vi "read_db.vi"(8 "error in (no error)":errorcluster, 11 "Constraints":T4={"Upper Timestamp Range"=timestamp(0 s since 1904-01-01), "Lower Timestamp Range"=timestamp(0 s since 1904-01-01), "Experiment Group:"="", "Experiment Name:"=[], "Upper Velocity Limit (km/s)"=0.0, "Lower Velocity Limit (km/s)"=0.0, "Upper Mass Limit (kg)"=0.0, "Lower Mass Limit (kg)"=0.0, "Estimate Source "=-2, "name array"=[]} {"Estimate Source" items=["Any Source."=-2, "No Shot"=-1, "Basic Labview Estimate"=0, "IDL Estimate From Andrew"=1, "IDL Estimate From Tobin"=2, "Old Metadata"=3]; "Lower Mass Limit (kg)" min=-1.0 max=1.0 step=1e-20; "Upper Mass Limit (kg)" min=-1.0 max=1.0 step=1e-20; "Lower Velocity Limit (km/s)" min=-1.0 max=299792000.0; "Upper Velocity Limit (km/s)" min=-1.0 max=299792000.0}) -> (0 "error out":errorcluster, 1 "Experiment Settings ID Array":i64[](array[numeric]), 2 "Dust Event ID Array":i64[](array[numeric]), 3 "Dust Array":T1[](array[typedef]) {"File Location" items=["Currently Writing"=-3, "Labview Files"=-2, "Mars Data Processing Factility"=-1, "Local Cache "=0, "Old Storage"=1, "Storage"=2]; "Estimate Source" items=["Any Source."=-2, "No Shot"=-1, "Basic Labview Estimate"=0, "IDL Estimate From Andrew"=1, "IDL Estimate From Tobin"=2, "Old Metadata"=3]}, 5 "File Location Array":i64[](array[numeric]))   [LabVIEW 2012]
uses:
  Constraints.ctl
  Estimate_source.ctl
  Public API/Query_Dust_Event.ctl
  File_location.ctl
  <vilib>/addons/database/Auxilliary.llb/DB Tools Cursor Type.ctl
  <vilib>/addons/database/Connection.llb/Conn Execute.vi
  <vilib>/addons/database/Recordset.llb/Rec Fetch Recordset Data (R).vi
  <vilib>/addons/database/Recordset.llb/Rec Destroy - Connection.vi
  <vilib>/addons/database/_DB Variant To Data/Database Variant To Data.xnode
  <vilib>/addons/database/NI_Database_API.lvlib
panel:
  out "concatenated string":string
  out "SQL Query Sintax":string
  # "Dust Event"
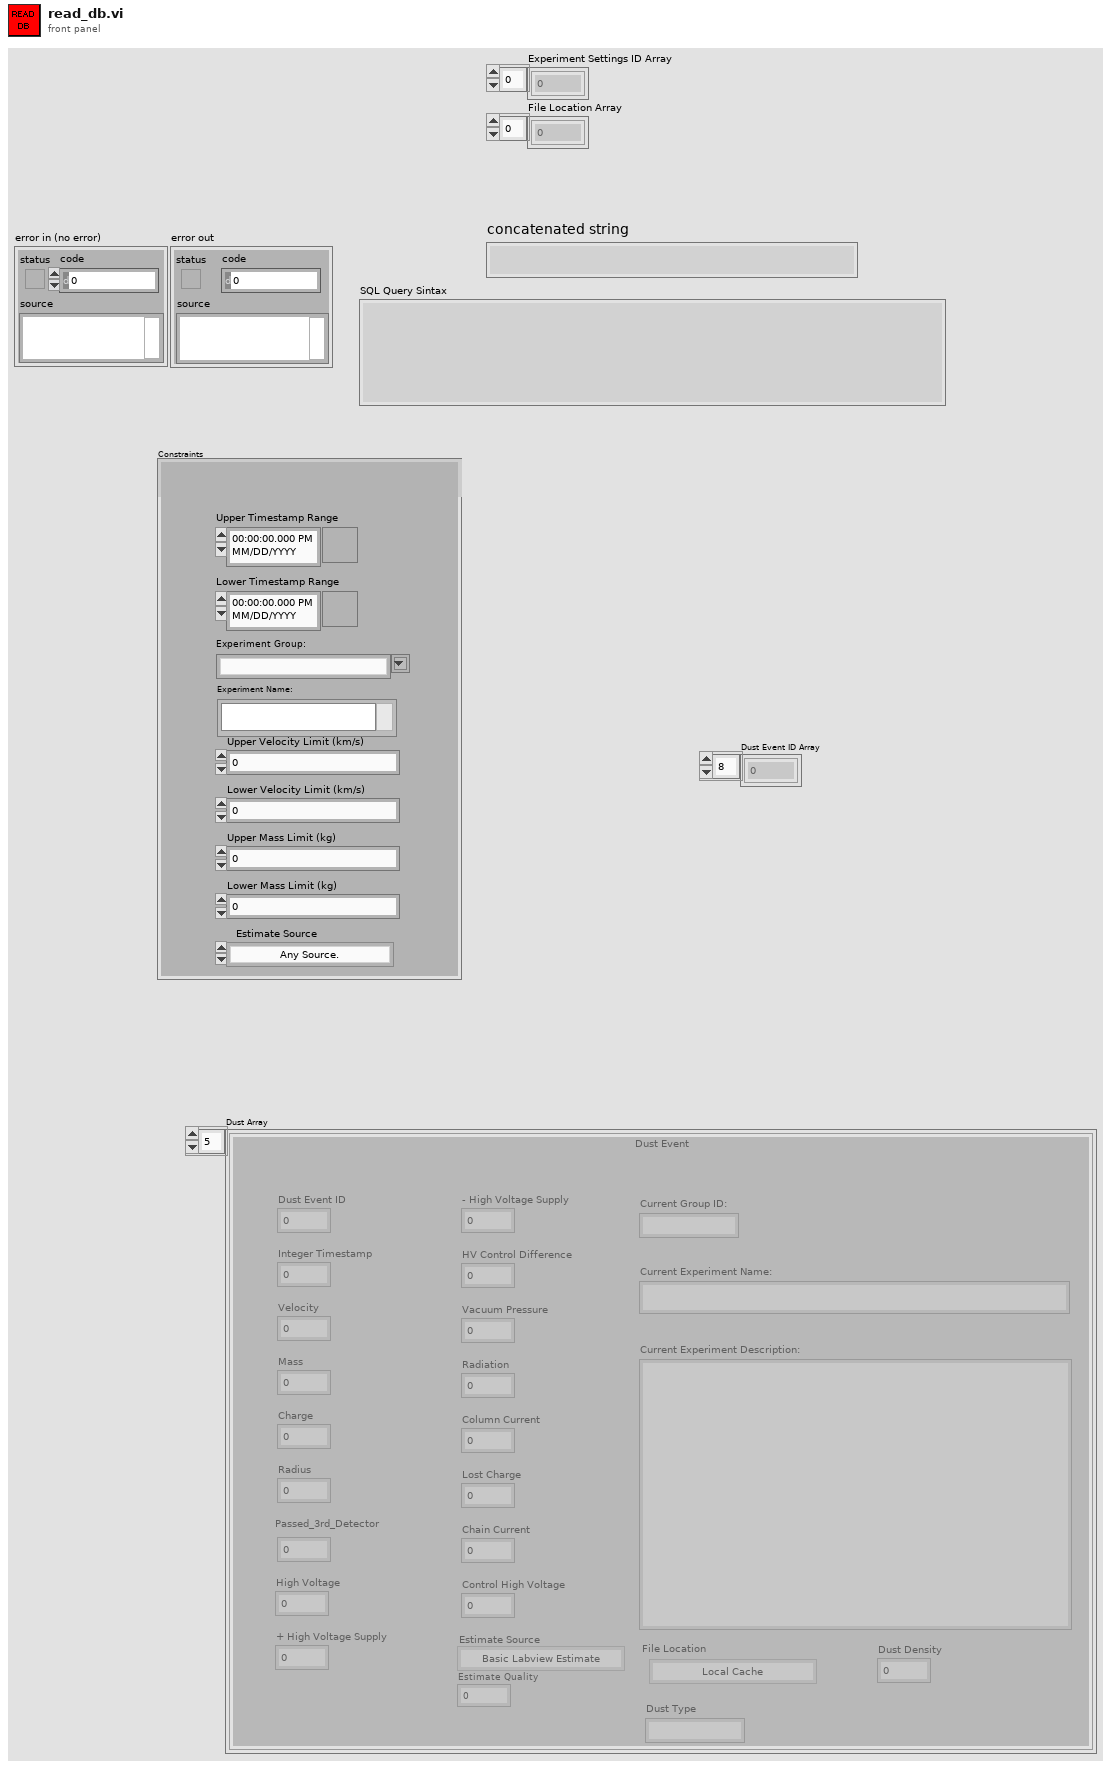
[diagram p1: front panel]
types:
  T1 = typedef "Query_Dust_Event.ctl" = cluster{"Dust Event ID":i64, "Integer Timestamp":i64, "Velocity":sgl, "Mass":sgl, "Charge":sgl, "Radius":sgl, "Passed_3rd_Detector":i8, "High Voltage":sgl, "+ High Voltage Supply":sgl, "- High Voltage Supply":sgl, "HV Control Difference":sgl, "Vacuum Pressure":sgl, "Radiation":sgl, "Column Current":sgl, "Lost Charge":sgl, "Chain Current":sgl, "Control High Voltage":sgl, "Current Group ID:":string, "Current Experiment Name:":string, "Current Experiment Description:":string, "Estimate Source":T2, "Estimate Quality":sgl, "File Location":T3, "Dust Type":string, "Dust Density":sgl}
  T2 = typedef "Estimate_source.ctl" = i8
  T3 = typedef "File_location.ctl" = i8
  T4 = typedef "Constraints.ctl" = cluster{"Upper Timestamp Range":timestamp, "Lower Timestamp Range":timestamp, "Experiment Group:":string, "Experiment Name:":i32[], "Upper Velocity Limit (km/s)":dbl, "Lower Velocity Limit (km/s)":dbl, "Upper Mass Limit (kg)":dbl, "Lower Mass Limit (kg)":dbl, "Estimate Source ":T2, "name array":string[]}
  T5 = typedef "NI_Database_API.lvlib/DB Tools Cursor Type.ctl" = enum16{"forward-only", "keyset", "dynamic", "static"}
  T6 = typedef "NI_Database_API.lvlib/Conn ObjectReference.ctl" = refnum<k1>
  T7 = typedef "NI_Database_API.lvlib/Rec ObjectReference.ctl" = refnum<k1>
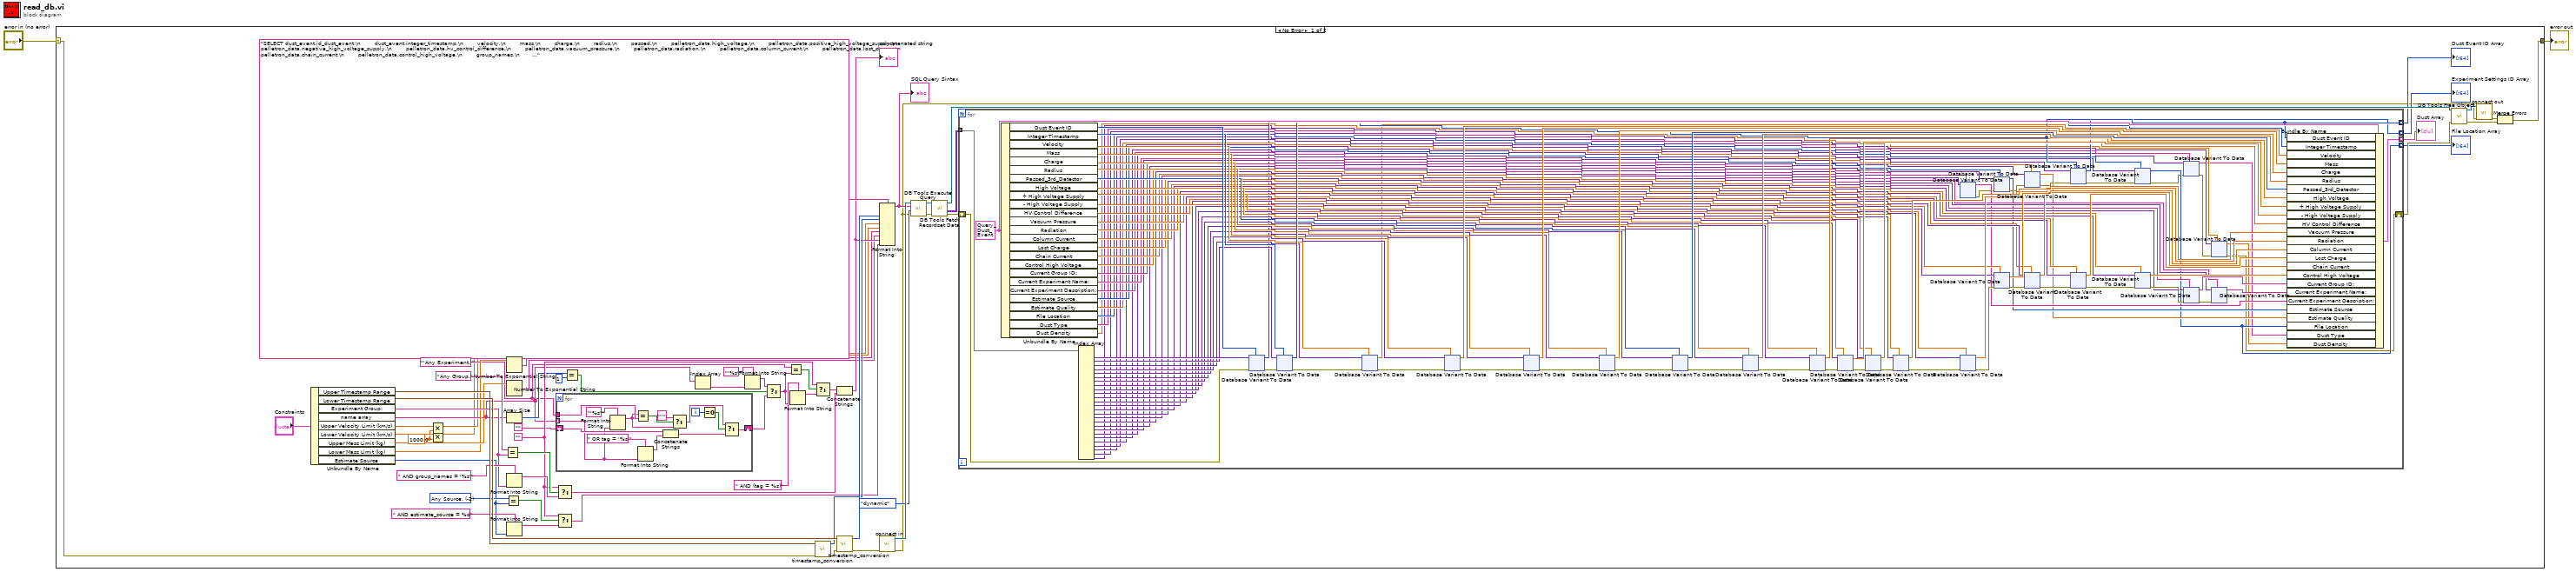
[diagram p0: block diagram]
diagram:
  n1 = case shown="No Error" "error in (no error)" {
    selector: "error in (no error)" -> [w57 w1020]
    tunnel: [w9 w1020] -> w1
    frame No Error {
      w3 = 1000.0 ("y")
      w26 = T2 -2 items=["Any Source."=-2, "No Shot"=-1, "Basic Labview Estimate"=0, "IDL Estimate From Andrew"=1, "IDL Estimate From Keith"=2, "Old Metadata"=3] ("Estimate Source")
      w21 = ""
      w13 = "'Any Experiment.'"
      n2 = Unbundle By Name("Constraints") -> ("Upper Timestamp Range"=w48:timestamp, "Lower Timestamp Range"=w49:timestamp, "Experiment Group:"=w43:string, "name array"=w14:string[], "Upper Velocity Limit (km/s)"=w33:dbl, "Lower Velocity Limit (km/s)"=w34:dbl, "Upper Mass Limit (kg)"=w32:dbl, "Lower Mass Limit (kg)"=w30:dbl, "Estimate Source"=w25:T2)
      n3 = Multiply(x=w33, y=w3) -> (x*y=w5:dbl)
      n4 = Multiply(x=w34, y=w3) -> (x*y=w4:dbl)
      n5 = Equal?(x="Any Group.", y=w43) -> (x = y?=w59:bool)
      n6 = Equal?(x=w26, y=w25) -> (x = y?=w24:bool)
      n7 = Number To Exponential String(number=w30) -> (E-format string=w29:string)  [unwired: 3 in]
      n8 = Number To Exponential String(number=w32) -> (E-format string=w31:string)  [unwired: 3 in]
      n9 = Array Size(array=w14) -> (size(s)=w20:i32)
      n10 = Format Into String(format string=" AND group_names = '%s'" ("string"), w43) -> (resulting string=w42:string)  [unwired: 2 in, 1 out]
      n11 = Format Into String(format string=" AND estimate_source = %d" ("string"), w25) -> (resulting string=w23:string)  [unwired: 2 in, 1 out]
      n12 = for {
        tunnel: w14 -> [w74] mode=indexing
        shift-right: [w76] -> w16
        shift-left: "" -> [w81]
        tunnel: w13 -> [w72]
        i -> [w78]
        n13 = Format Into String(format string="'%s'", w74) -> (resulting string=w70:string)  [unwired: 2 in, 1 out]
        n14 = Equal?(x=w70, y=w72) -> (x = y?=w71:bool)
        n15 = Format Into String(format string=" OR tag = '%s'" ("string"), w74) -> (resulting string=w80:string)  [unwired: 2 in, 1 out]
        n16 = Concatenate Strings(w81, w80) -> (w75:string)
        n17 = Select(t="''", s=w71, f=w70) -> (s? t:f=w69:string)
        n18 = Equal To 0?(x=w78) -> (x = 0?=w77:bool)
        n19 = Select(t=w69, s=w77, f=w75) -> (s? t:f=w76:string)
      }
      n20 = Select(t=w21, s=w59, f=w42) -> (s? t:f=w54:string)
      n21 = Select(t=w21, s=w24, f=w23) -> (s? t:f=w22:string)
      n22 = Equal?(x=w20, y=1) -> (x = y?=w18:bool)
      n23 = Index Array(array=w14) -> (element=w12:string)  [unwired: 1 in]
      n24 = Format Into String(format string="'%s'", w12) -> (resulting string=w11:string)  [unwired: 2 in, 1 out]
      n25 = Select(t=w11, s=w18, f=w16) -> (s? t:f=w17:string)
      n26 = Equal?(x=w13, y=w17) -> (x = y?=w60:bool)
      n27 = Format Into String(format string=" AND (tag = %s)" ("string"), w17) -> (resulting string=w40:string)  [unwired: 2 in, 1 out]
      n28 = Select(t=w21, s=w60, f=w40) -> (s? t:f=w55:string)
      n29 = call "timestamp_conversion.vi"("error in (no error)"=w57, "Time Stamp"=w48) -> ("error out"=w58:errorcluster, "Integer Time"=w38:i64)  [unwired: 7 in]
      n30 = Concatenate Strings(w55, w54) -> (w35:string)
      "concatenated string" <- w35
      n31 = call "timestamp_conversion.vi"("error in (no error)"=w58, "Time Stamp"=w49) -> ("error out"=w51:errorcluster, "Integer Time"=w39:i64)  [unwired: 7 in]
      n32 = Format Into String(format string="SELECT dust_event.id_dust_event,\n        dust_event.integer_timestamp,\n        velocity,\n        mass,\n        charge,\n        radius,\n        passed,\n        pelletron_data.high_voltage,\n        pelletron_data.positive_high_voltage_supply,\n        pelletron_data.negative_high_voltage_supply,\n        pelletron_data.hv_control_difference,\n        pelletron_data.vacuum_pressure,\n        pelletron_data.radiation,\n        pelletron_data.column_current,\n        pelletron_data.lost_charge,\n        pelletron_data.chain_current,\n        pelletron_data.control_high_voltage,\n        group_names,\n        tag,\n        description,\nestimate_source, \nestimate_quality,\ndust_event.id_experiment_settings,\ndust_event.file_location,\ndust_type.dust_name,\ndust_type.dust_density\n\nFROM\n    dust_event\n        INNER JOIN \n    experiment_settings ON dust_event.id_experiment_settings = experiment_settings.id_experiment_settings\n        INNER JOIN  \n    groups ON experiment_settings.id_groups=groups.id_groups\n        INNER JOIN\n    pelletron_data ON pelletron_data.id_pelletron_data = dust_event.id_pelletron_data\nINNER JOIN\n     dust_info ON dust_event.id_dust_info = dust_info.id_dust_info\n\t\tINNER join\n\tdust_type ON dust_info.dust_type = dust_type.id_dust_type\n\nWHERE dust_event.integer_timestamp >= %d  AND dust_event.integer_timestamp <= %d AND dust_event.velocity >= %d  AND dust_event.velocity <= %d AND dust_event.mass >= %s  AND dust_event.mass <= %s%s%s\nORDER BY dust_event.integer_timestamp; " ("string"), w39, w38, w4, w5, w29, w31, w35, w22) -> (resulting string=w36:string)  [unwired: 2 in, 1 out]
      "SQL Query Sintax" <- w36
      n33 = call "connect in.vi"("error in (no error)"=w51) -> ("error out"=w6:errorcluster, "Database Connection"=w62:T6)  [unwired: 6 in, 1 out]
      n34 = call-poly <vilib>:"DB Tools Execute Query.vi"("error in (no error)"=w6, "cursor type"=DB_Tools_Cursor_Type."dynamic", "SQL query"=w36, "connection reference"=w62) -> ("error out"=w66:errorcluster, "recordset reference"=w67:T7)  [unwired: 4 in]
      n35 = call-poly <vilib>:"DB Tools Fetch Recordset Data.vi"("error in (no error)"=w66, "recordset reference"=w67) -> ("error out"=w64:errorcluster, "recordset data"=w53:variant[][], "recordset reference out"=w65:T7)  [unwired: 3 in]
      n36 = for {
        tunnel: w53 -> [w187] mode=indexing
        shift-right: [w85] -> w63
        shift-left: w64 -> [w186]
        tunnel: [w108] -> w52 mode=indexing
        tunnel: [w98] -> w46 mode=indexing
        tunnel: [w96] -> w45 mode=indexing
        tunnel: [w92] -> w28 mode=indexing
        w183 = T1 {"Dust Event ID"=0, "Integer Timestamp"=0, "Velocity"=0.0, "Mass"=0.0, "Charge"=0.0, "Radius"=0.0, "Passed_3rd_Detector"=0, "High Voltage"=0.0, "+ High Voltage Supply"=0.0, "- High Voltage Supply"=0.0, "HV Control Difference"=0.0, "Vacuum Pressure"=0.0, "Radiation"=0.0, "Column Current"=0.0, "Lost Charge"=0.0, "Chain Current"=0.0, "Control High Voltage"=0.0, "Current Group ID:"="", "Current Experiment Name:"="", "Current Experiment Description:"="", "Estimate Source"=0, "Estimate Quality"=0.0, "File Location"=0, "Dust Type"="", "Dust Density"=0.0} ("Cluster")
        n37 = Unbundle By Name(w183) -> ("Dust Event ID"=w185:i64, "Integer Timestamp"=w181:i64, "Velocity"=w177:sgl, "Mass"=w174:sgl, "Charge"=w171:sgl, "Radius"=w166:sgl, "Passed_3rd_Detector"=w162:i8, "High Voltage"=w158:sgl, "+ High Voltage Supply"=w153:sgl, "- High Voltage Supply"=w150:sgl, "HV Control Difference"=w145:sgl, "Vacuum Pressure"=w141:sgl, "Radiation"=w137:sgl, "Column Current"=w133:sgl, "Lost Charge"=w129:sgl, "Chain Current"=w125:sgl, "Control High Voltage"=w121:sgl, "Current Group ID:"=w117:string, "Current Experiment Name:"=w113:string, "Current Experiment Description:"=w110:string, "Estimate Source"=w104:T2, "Estimate Quality"=w103:sgl, "File Location"=w93:T3, "Dust Type"=w90:string, "Dust Density"=w89:sgl)
        n38 = Index Array(array=w187) -> (element #1=w184:variant, element #2=w182:variant, element #3=w178:variant, element #4=w175:variant, element #5=w170:variant, element #6=w165:variant, element #7=w163:variant, element #8=w159:variant, element #9=w155:variant, element #10=w151:variant, element #11=w146:variant, element #12=w142:variant, element #13=w138:variant, element #14=w135:variant, element #15=w130:variant, element #16=w126:variant, element #17=w122:variant, element #18=w118:variant, element #19=w114:variant, element #20=w109:variant, element #21=w102:variant, element #22=w101:variant, element #23=w99:variant, element #24=w94:variant, element #25=w88:variant, element #26=w87:variant)  [unwired: 26 in]
        n39 = xnode "Database Variant To Data"("database variant"=w184, "error in"=w186, "type"=w185) -> ("data"=w98:i64, "error out"=w179:errorcluster)
        n40 = xnode "Database Variant To Data"("database variant"=w182, "error in"=w179, "type"=w181) -> ("data"=w180:i64, "error out"=w176:errorcluster)
        n41 = xnode "Database Variant To Data"("database variant"=w178, "error in"=w176, "type"=w177) -> ("data"=w82:sgl, "error out"=w172:errorcluster)
        n42 = xnode "Database Variant To Data"("database variant"=w175, "error in"=w172, "type"=w174) -> ("data"=w173:sgl, "error out"=w168:errorcluster)
        n43 = xnode "Database Variant To Data"("database variant"=w170, "error in"=w168, "type"=w171) -> ("data"=w169:sgl, "error out"=w167:errorcluster)
        n44 = xnode "Database Variant To Data"("database variant"=w165, "error in"=w167, "type"=w166) -> ("data"=w164:sgl, "error out"=w160:errorcluster)
        n45 = xnode "Database Variant To Data"("database variant"=w163, "error in"=w160, "type"=w162) -> ("data"=w161:i8, "error out"=w156:errorcluster)
        n46 = xnode "Database Variant To Data"("database variant"=w159, "error in"=w156, "type"=w158) -> ("data"=w157:sgl, "error out"=w154:errorcluster)
        n47 = xnode "Database Variant To Data"("database variant"=w155, "error in"=w154, "type"=w153) -> ("data"=w152:sgl, "error out"=w148:errorcluster)
        n48 = xnode "Database Variant To Data"("database variant"=w151, "error in"=w148, "type"=w150) -> ("data"=w149:sgl, "error out"=w147:errorcluster)
        n49 = xnode "Database Variant To Data"("database variant"=w146, "error in"=w147, "type"=w145) -> ("data"=w144:sgl, "error out"=w143:errorcluster)
        n50 = xnode "Database Variant To Data"("database variant"=w142, "error in"=w143, "type"=w141) -> ("data"=w140:sgl, "error out"=w139:errorcluster)
        n51 = xnode "Database Variant To Data"("database variant"=w109, "type"=w110) -> ("data"=w111:string, "error out"=w106:errorcluster)  [unwired: 1 in]
        n52 = xnode "Database Variant To Data"("database variant"=w138, "error in"=w139, "type"=w137) -> ("data"=w136:sgl, "error out"=w134:errorcluster)
        n53 = xnode "Database Variant To Data"("database variant"=w102, "error in (no error)"=w106, "type"=w104) -> ("data"=w107:T2, "error out"=w105:errorcluster)
        n54 = xnode "Database Variant To Data"("database variant"=w135, "error in"=w134, "type"=w133) -> ("data"=w132:sgl, "error out"=w131:errorcluster)
        n55 = xnode "Database Variant To Data"("database variant"=w101, "error in"=w105, "type"=w103) -> ("data"=w100:sgl, "error out"=w97:errorcluster)
        n56 = xnode "Database Variant To Data"("database variant"=w130, "error in"=w131, "type"=w129) -> ("data"=w128:sgl, "error out"=w127:errorcluster)
        n57 = xnode "Database Variant To Data"("database variant"=w99, "error in"=w97, "type"=w98) -> ("data"=w96:i64, "error out"=w95:errorcluster)
        n58 = xnode "Database Variant To Data"("database variant"=w126, "error in"=w127, "type"=w125) -> ("data"=w124:sgl, "error out"=w123:errorcluster)
        n59 = xnode "Database Variant To Data"("database variant"=w94, "error in (no error)"=w95, "type"=w93) -> ("data"=w92:T3, "error out"=w86:errorcluster)
        n60 = xnode "Database Variant To Data"("database variant"=w122, "error in"=w123, "type"=w121) -> ("data"=w120:sgl, "error out"=w119:errorcluster)
        n61 = xnode "Database Variant To Data"("database variant"=w88, "error in"=w86, "type"=w90) -> ("data"=w84:string, "error out"=w91:errorcluster)
        n62 = xnode "Database Variant To Data"("database variant"=w118, "error in"=w119, "type"=w117) -> ("data"=w116:string, "error out"=w115:errorcluster)
        n63 = xnode "Database Variant To Data"("database variant"=w87, "error in"=w91, "type"=w89) -> ("data"=w83:sgl, "error out"=w85:errorcluster)
        n64 = xnode "Database Variant To Data"("database variant"=w114, "error in"=w115, "type"=w113) -> ("data"=w112:string)  [unwired: 1 out]
        n65 = Bundle By Name(cluster=w183, "Dust Event ID"=w98, "Integer Timestamp"=w180, "Velocity"=w82, "Mass"=w173, "Charge"=w169, "Radius"=w164, "Passed_3rd_Detector"=w161, "High Voltage"=w157, "+ High Voltage Supply"=w152, "- High Voltage Supply"=w149, "HV Control Difference"=w144, "Vacuum Pressure"=w140, "Radiation"=w136, "Column Current"=w132, "Lost Charge"=w128, "Chain Current"=w124, "Control High Voltage"=w120, "Current Group ID:"=w116, "Current Experiment Name:"=w112, "Current Experiment Description:"=w111, "Estimate Source"=w107, "Estimate Quality"=w100, "File Location"=w92, "Dust Type"=w84, "Dust Density"=w83) -> (w108:T1)
      }
      "Dust Array" <- w52
      "Dust Event ID Array" <- w46
      "Experiment Settings ID Array" <- w45
      "File Location Array" <- w28
      n66 = call-poly <vilib>:"DB Tools Free Object.vi"("error in (no error)"=w63, "recordset reference"=w65) -> ("error out"=w7:errorcluster, "connection reference"=w61:T6)  [unwired: 8 in]
      n67 = call "connect out.vi"("error in (no error)"=w6, "connection reference"=w61) -> ("error out"=w8:errorcluster)  [unwired: 9 in]
      n68 = Merge Errors(w8, w7) -> (w9:errorcluster)
    }
    frame Error {
    }
  }
  "error out" <- w1
